vi "CIC Filter.vi"(0 "input data":fxp<+/-,20,5>, 7 "sample":bool=TRUE, 9 "input valid":bool) -> (4 "output data":fxp<+/-,20,5>=-16.0, 10 "output valid":bool=TRUE, 14 "ready for input":bool=TRUE)   [LabVIEW 2011]
doc: "----------------------\n\nThis filter is configured as follows:\n\n<b>Filter Configuration</b>\nType: Multirate - Decimation\nStructure: CIC\nNumber of stages: 2\nDifferential delay: 1\nFactor: 32\n\n<b>Input Data Type</b>\nType: fixed-point <±,20,5> [-1.600000E+1,1.599997E+1]:3.051758E-5\n\n<b>Output Data Type</b>\nType: fixed-point <±,20,5> [-1.600000E+1,1.599997E+1]:3.051758E-5\nRounding mode: Round-Half-Even\nOverflow mode: Saturate\n\n<b>Implementation</b>\nNumber of channels: 1\nMaximum input sampling rate per channel @ 40MHz: 40MHz\nGain processing: On Host\n\n<b>Execution Mode</b>\nInside single-cycle Timed Loop\nThroughput: 1 cycle/sample\n\n<b>Estimated Resources</b>\nLUT: 118"
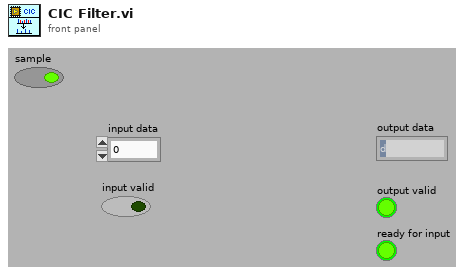
[diagram p1: front panel]
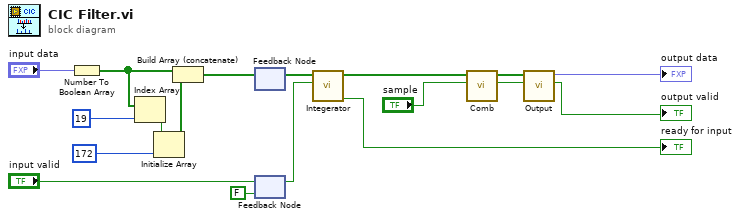
[diagram p0: block diagram]
diagram:
  n1 = Number To Boolean Array(number="input data") -> (Boolean array=w18:bool[])
  n2 = Index Array(array=w18, index=19 ("input msb")) -> (element=w10:bool)
  n3 = Initialize Array(w10, 172 ("192-input wl")) -> (w12:bool[])
  n4 = Build Array (concatenate)(w18, w12) -> (w16:bool[])
  n5 = feedback-in #1(w16) -> ()
  n6 = feedback #1() -> (w7:bool[])  [unwired: 1 out]
  n7 = feedback-in #2("input valid") -> ()
  n8 = feedback #2(FALSE ("input valid")) -> (w6:bool)
  n9 = call "Integerator.vi"("input valid"=w6, "data in"=w7) -> ("ready for input"=→"ready for input":bool, "data out"=w4:bool[])  [unwired: 7 in, 1 out]
  n10 = call "Comb.vi"("sample"="sample", "data in"=w4) -> ("output valid"=w8:bool, "data out"=w9:bool[])  [unwired: 7 in, 1 out]
  n11 = call "Output.vi"("input valid"=w8, "input data"=w9) -> ("output valid"=→"output valid":bool, "output data"=→"output data":fxp<+/-,20,5>)  [unwired: 8 in]
